vi "NanotecSMCPD.find axis reference.vi"(0 "i ref in":refnum<vi>, 1 "axis":i32, 3 "ms timeout (10000)":i32=10000, 5 "error in (no error)":errorcluster) -> (14 "i ref out":refnum<vi>, 17 "timed out":bool, 19 "error out":errorcluster)   [LabVIEW 2014, in "NanotecSMCPD.lvlib"]
doc: "References an axis by moving to the negative limit switch. The controller will gently stop the motion and move back to the motion when the switch was touched.\n\nThis method just initiates the reference move. Use the method \"check axis reference move\" to determine, if the operation was successful."
uses:
  NanotecSMCPD.lvlib
  CS_Core/CSSystem/CoreDefs/CoreDefs.error_type.ctl
  CS_Core/CSSystem/CoreDefs/CoreDefs.error_severity.ctl
  CS_Core/CSApplicationBaseClasses/MotorBase/MotorBase.statusType.ctl
  CS_Core/CSApplicationBaseClasses/MotorBase/MotorBase.directionType.ctl
  CS_Core/CSApplicationBaseClasses/MotorBase/MotorBase.serviceType.ctl
  CSlibraries/UtilityLib/UtilityLib.valueStatus.ctl
  CS_Core/CSApplicationBaseClasses/DeviceBase/DeviceBase.lvlib
  CS_Core/CSSystem/CoreLib/CoreLib.lvlib
  CS_Core/CSApplicationBaseClasses/MotorBase/MotorBase.lvlib
  instr.lib/NanotecSMCPD/NanotecSMCPDDriver.lvlib
  CSlibraries/UtilityLib/UtilityLib.lvlib
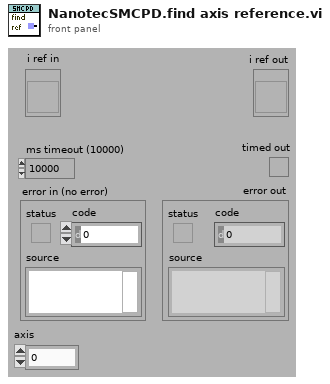
[diagram p1: front panel]
types:
  T1 = typedef "CoreDefs.error_severity.ctl" = enum16{"undefined", "information", "warning", "error", "fatal"}
  T2 = typedef "CoreDefs.error_type.ctl" = enum16{"no error", "can't load process", "can't unload process", "process does not exist", "can't install process", "can't remove process", "unknown function", "time out", "can't execute function", "duplicate queue name", "super not found", "caller queue invalid", "can't ping process", "unknown error", "VISA Error", "VISA timeout", "GPIB timeout", "GPIB error", "communication error", "data type mismatch", "can't read data from OPC server", "can't write data to OPC server", "OET error", "function not implemented", "process already exists", "invalid Shared Variable name", "error writing Shared Variable", "error reading Shared Variable", "invalid client name", "corrupt database", "unknown class", "call not authorized", "parameter out of range", "OET timeout: can't get data to modify", "invalid queue name", "requested operation incompatible with current state", "event undefined", "event disabled", "state undefined", "caller is not a friend", "EventBuilder: bad eventID", "EventBuilder: no DAQ devices", "a thread must not stop itself", "UNUSED ELEMENT4", "DiscArchiver: eventData incomplete", "DiscArchiver: eventData does not belong to run", "DiscArchiver: can't open file", "DiscArchiver: can't write to file", "DiscArchiver: available disc space low", "can't acquire semaphore", "error reading data from database", "notifier object is not existing", "can't register process", "can't unregister process", "illegal event type", "object disabled", "object already exists", "can't change state", "Instrument not found", "no connection to remote node", "invalid reference", "N/A", "UNUSED ELEMENT 1", "element not found", "illegal TCP/IP connection detected", "object does not exist", "invalid access ID", "unknown CS system", "invalid privilige", "unsupported data type", "unsupported server type", "IO server already exists", "Shared Variable already exists"}
  T3 = typedef "UtilityLib.lvlib/UtilityLib.valueStatus.ctl" = enum16{"no info available", "stand by/off", "on", "warning", "alarm/malfunction", "not implemented", "user action required", "important information", "system default", "control default", "indicator default", "button default"}
  T4 = typedef "MotorBase.lvlib/MotorBase.serviceType.ctl" = enum16{"onOff", "startVelocity", "stopVelocity", "acceleration", "rangeMin", "rangeMax", "status", "position"}
  T5 = typedef "MotorBase.lvlib/MotorBase.directionType.ctl" = enum16{"unknown", "update actual value", "update nominal value", "update both"}
  T6 = typedef "MotorBase.lvlib/MotorBase.statusType.ctl" = u32
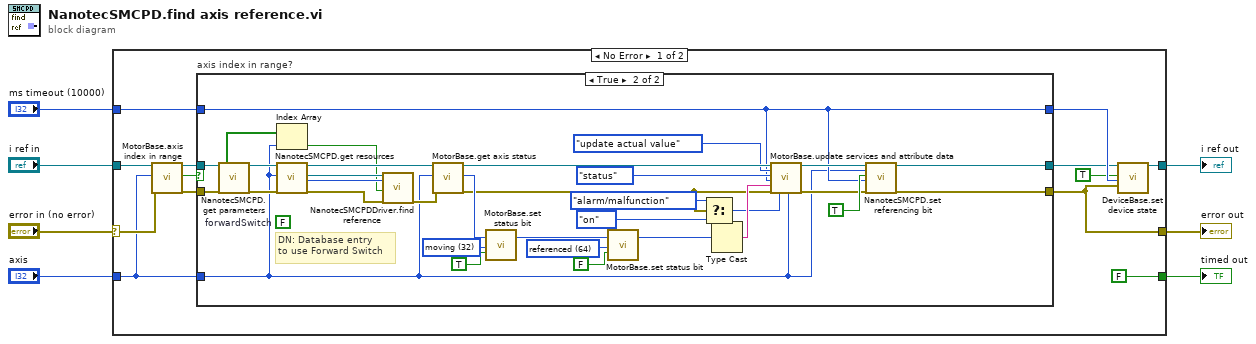
[diagram p0: block diagram]
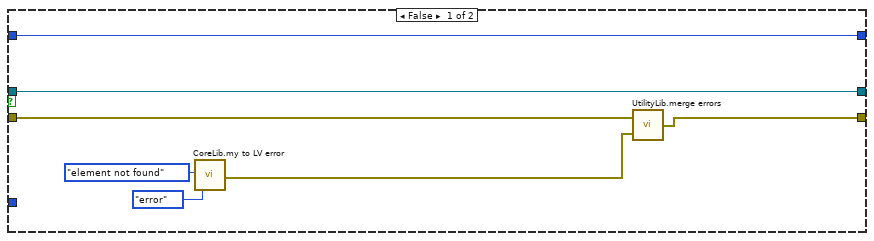
[diagram p2: hidden frame]
diagram:
  n1 = case shown="No Error" "error in (no error)" {
    selector: "error in (no error)" -> [w13 w61]
    tunnel: "ms timeout (10000)" -> [w10 _]
    tunnel: "i ref in" -> [w14 w62]
    tunnel: [w12 w61] -> w4
    tunnel: "axis" -> [w11 _]
    tunnel: [w9 w62] -> w2
    tunnel: [FALSE _] -> w1
    frame No Error {
      n2 = call "MotorBase.axis index in range.vi"("i ref in"=w14, "axisIndex"=w11, "error in (no error)"=w13) -> ("i ref out"=w18:refnum<vi>, "in range"=w17:bool, "error out"=w19:errorcluster)  [unwired: 14 in]
      n3 = case "axis index in range?" shown="True" w17 {
        tunnel: [w27 w28] -> w16
        tunnel: [w21 w29] -> w12
        tunnel: w10 -> [w24 w43]
        tunnel: w11 -> [_ w30]
        tunnel: w18 -> [w27 w35]
        tunnel: w19 -> [w23 w34]
        tunnel: [w24 w43] -> w20
        frame False {
          n4 = call "CoreLib.my to LV error.vi"("ErrorTypes"=CoreDefs.error_type."element not found", "severityLevel"=CoreDefs.error_severity."error") -> ("myErrorCluster"=w22:errorcluster)  [unwired: 16 in, 1 out]
          n5 = call "UtilityLib.merge errors.vi"("error2 (no error)"=w22, "error1 (no error)"=w23) -> ("error out"=w21:errorcluster)
        }
        frame True {
          w50 = T6 64 items=["motorEnabled"=1, "negativeLimitSwitchActive"=2, "positiveLimitSwitchActive"=4, "limitSwitchesEnabled"=8, "limitSwitchesAreNormallyClosed"=16, "moving"=32, "referenced"=64, "inPosition"=128, "reserved2"=256, "reserved3"=512, "reserved4"=1024, "reserved5"=2048, "error"=4096, "reserved6"=8192, "reserved7"=16384, "reserved8"=32768, "user defined1"=65536, "user defined2"=131072, "user defined3"=262144, "user defined4"=524288, "user defined5"=1048576, "user defined6"=2097152, "user defined7"=4194304, "user defined8"=8388608, "user defined9"=16777216, "user defined10"=33554432, "user defined11"=67108864, "user defined12"=134217728, "user defined13"=268435456, "user defined14"=536870912, "user defined15"=1073741824, "user defined16"=2147483648] ("statusBit")
          w53 = T6 32 items=["motorEnabled"=1, "negativeLimitSwitchActive"=2, "positiveLimitSwitchActive"=4, "limitSwitchesEnabled"=8, "limitSwitchesAreNormallyClosed"=16, "moving"=32, "referenced"=64, "inPosition"=128, "reserved2"=256, "reserved3"=512, "reserved4"=1024, "reserved5"=2048, "error"=4096, "reserved6"=8192, "reserved7"=16384, "reserved8"=32768, "user defined1"=65536, "user defined2"=131072, "user defined3"=262144, "user defined4"=524288, "user defined5"=1048576, "user defined6"=2097152, "user defined7"=4194304, "user defined8"=8388608, "user defined9"=16777216, "user defined10"=33554432, "user defined11"=67108864, "user defined12"=134217728, "user defined13"=268435456, "user defined14"=536870912, "user defined15"=1073741824, "user defined16"=2147483648] ("statusBit")
          (unwired) FALSE  # forwardSwitch
          # "DN: Database entry\nto use Forward Switch"
          n6 = call "NanotecSMCPD.get parameters.vi"("i ref in"=w35, "error in (no error)"=w34) -> ("ReverseDirection?"=w32:bool[], "i ref out"=w36:refnum<vi>, "error out"=w33:errorcluster)  [unwired: 6 in, 9 out]
          n7 = Index Array(array=w32, index=w30) -> (element=w31:bool)
          n8 = call "NanotecSMCPD.get resources.vi"("i ref in"=w36, "axisNumber"=w30, "error in (no error)"=w33) -> ("i ref out"=w56:refnum<vi>, "VISA resource"=w60:refnum<visa-resource-name>, "address"=w59:i32, "error out"=w58:errorcluster)  [unwired: 13 in]
          n9 = call "NanotecSMCPDDriver.find reference.vi"("VISA resource name"=w60, "contollerID"=w59, "forwardSwitch"=w31, "error in (no error)"=w58) -> ("error out"=w55:errorcluster)  [unwired: 13 in, 2 out]
          n10 = call "MotorBase.get axis status.vi"("i ref in"=w56, "axisIndex"=w30, "error in (no error)"=w55) -> ("i ref out"=w48:refnum<vi>, "status"=w54:T6, "error out"=w40:errorcluster)  [unwired: 14 in]
          n11 = call "MotorBase.set status bit.vi"("status"=w54, "statusBit"=w53, "setBit"=TRUE) -> ("status out"=w51:T6)  [unwired: 16 in]
          n12 = call "MotorBase.set status bit.vi"("status"=w51, "statusBit"=w50, "setBit"=FALSE) -> ("status out"=w42:T6)  [unwired: 16 in]
          n13 = Select(t=UtilityLib.valueStatus."alarm/malfunction", s=w40, f=UtilityLib.valueStatus."on" ("quality")) -> (s? t:f=w37:T3)
          n14 = Type Cast(x=w42) -> (*(type *) &x=w41:string)  [unwired: 1 in]
          n15 = call "MotorBase.update services and attribute data.vi"("i ref in"=w48, "direction"=MotorBase.directionType."update actual value", "service"=MotorBase.serviceType."status", "ms timeout (10000)"=w43, "value"=w41, "error in (no error)"=w40, "quality"=w37, "axisNumber"=w30) -> ("i ref out"=w46:refnum<vi>, "error out"=w47:errorcluster)  [unwired: 9 in, 1 out]
          n16 = call "NanotecSMCPD.set referencing bit.vi"("i ref in"=w46, "axis"=w30, "isReferencing?"=TRUE ("referencing?"), "ms timeout (10000)"=w43, "error in (no error)"=w47) -> ("i ref out"=w28:refnum<vi>, "error out"=w29:errorcluster)  [unwired: 12 in, 1 out]
        }
      }
      n17 = call "DeviceBase.set device state.vi"("i ref in"=w16, "implicit"=TRUE, "ms timeout (10000)"=w20, "device error"=w12) -> ("i ref out"=w9:refnum<vi>)  [unwired: 13 in, 2 out]
    }
    frame Error {
    }
  }
  "error out" <- w4
  "i ref out" <- w2
  "timed out" <- w1
